vi "7118ValveCntrl.vi"() -> ()   [LabVIEW 2017]
doc: "Manually blink and LED attached to a digital output channel of a LINX device by clicking and LED control in LabVIEW."
uses:
  <vilib>/MakerHub/LINX/Public/Peripherals/Digital/Digital Write N Chans.vi
  <vilib>/MakerHub/LINX/Private/Local IO/LinxDigitalWrite.vi
  <vilib>/MakerHub/LINX/Public/Utilities/Check Channel.vi
  <vilib>/MakerHub/LINX/Public/Utilities/Open Serial.vi
  <vilib>/MakerHub/LINX/Private/Utilties/Generate Error.vi
  <vilib>/MakerHub/LINX/LMH-LINX.lvlib
panel:
  in  "Boolean":bool
  in  "device ID":u32 format="%.0x"
  in  "CHANNELS":u8[](array[numeric])
  out "Loop Rate (Hz)":u32
  in  "MANUAL CONTROLS":bool[](array[boolean])
  in  "Serial Port":refnum<visa-resource-name>
  in  "Stop Button":bool
  # "VALVE CONTROL\nVALVE CONTROl\nVALVE CONTROL\nVLV CNTRL"
  # "MCU Control"
  # "OPERATOR INSTRUCTIONS - MCU \n\n1. LOAD FIRMWARE ONTO MCU\n2. SELECT COM PORT\n3. SELECT ALL CHANNELS/CORRESPONDING TO MCU PIN NUMBERS\n4. RUN THE SCRIPT - WAIT 10-15 SECOND TO INITIALIZE  \n5. IF INITILIAZATION ERROR RECEIVED - RUN THE SCRIPT AGAIN\n6. CONTROLS ARE READY WHEN THE HZ RATE SETTLES"
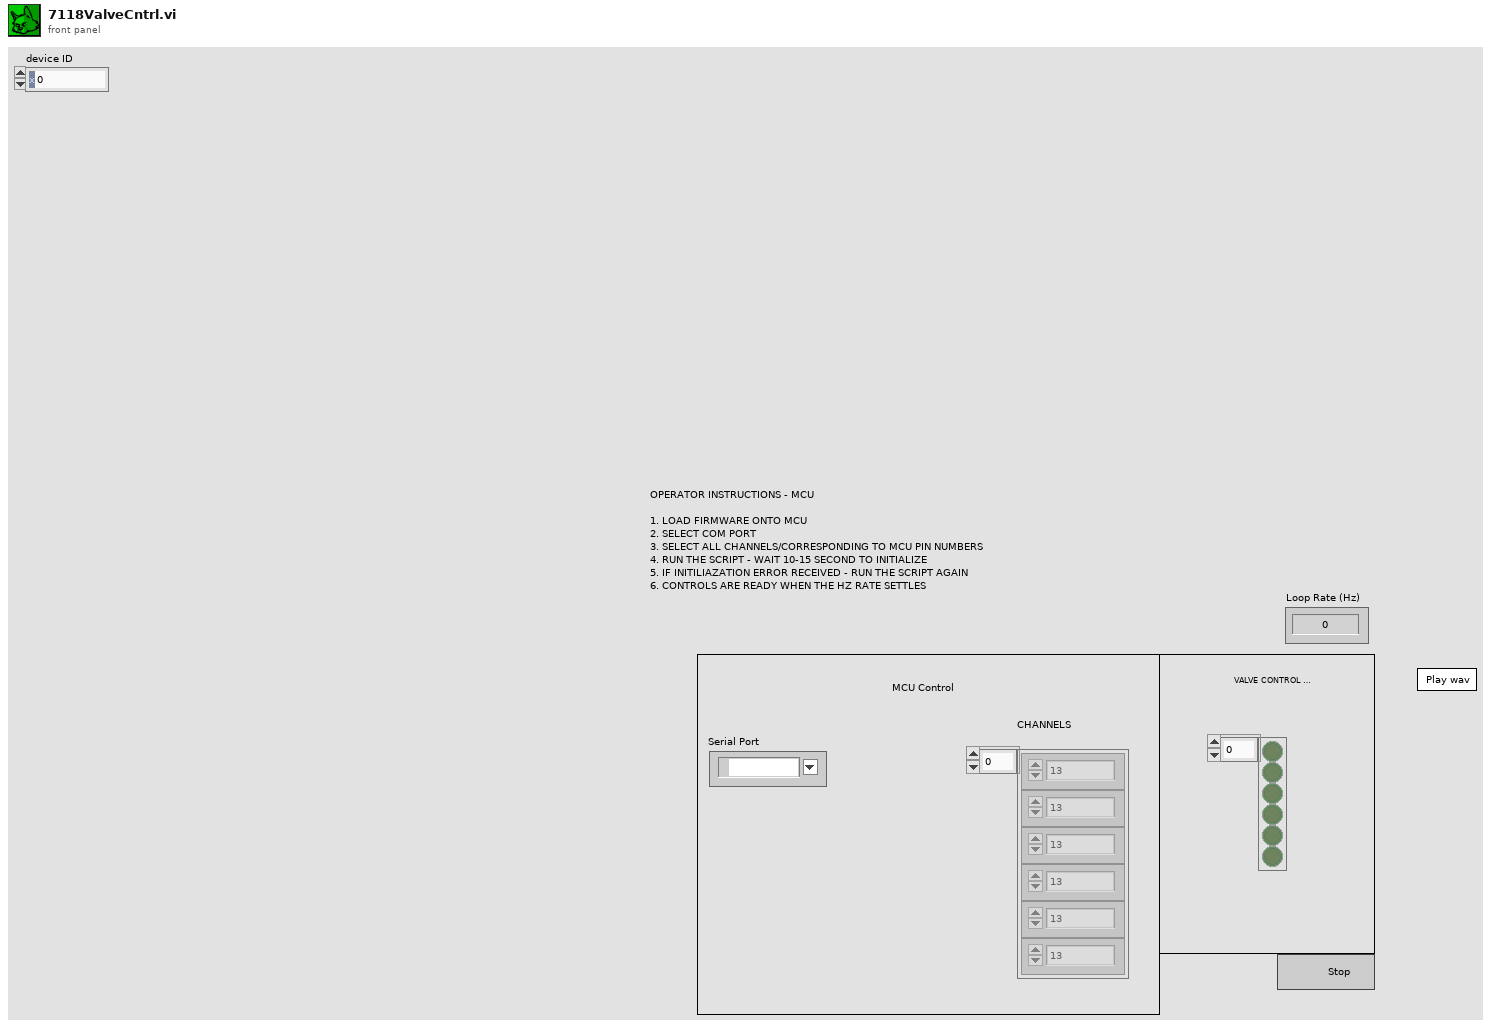
[diagram p1: front panel]
types:
  T1 = typedef "LMH-LINX.lvlib/LINX Ref.ctl" = cluster{"IO":T2, "Interface":T3, "LINX Device Config":T4}
  T2 = typedef "LMH-LINX.lvlib/Platform.ctl" = enum16{"Remote", "Local"}
  T3 = typedef "LMH-LINX.lvlib/Interface.ctl" = enum16{"Serial", "TCP"}
  T4 = typedef "LMH-LINX.lvlib/Device.lvlib/LINX Device Config.ctl" = cluster{"Interface":T3, "COM Port":refnum<visa-resource-name>, "TCP Configuration":T5, "Device Family":u8, "Device ID":u8, "Device Name":string, "TCP Ref":refnum<k5>, "Channels":T6}
  T5 = typedef "LMH-LINX.lvlib/Device.lvlib/TCP Config.ctl" = cluster{"IP Address":string, "Port":u16}
  T6 = typedef "LMH-LINX.lvlib/Channels.ctl" = cluster{"DI":u8[], "DO":u8[], "AI":u8[], "AO":u8[], "PWM":u8[], "QE":u8[], "UART":u8[], "I2C 2":u8[], "SPI":u8[], "CAN":u8[], "Servo":u8[], "AI Ref (V)":dbl, "AI Resolution (Bits)":u8, "AO Ref (V)":dbl, "AO Resolution (Bits)":u8}
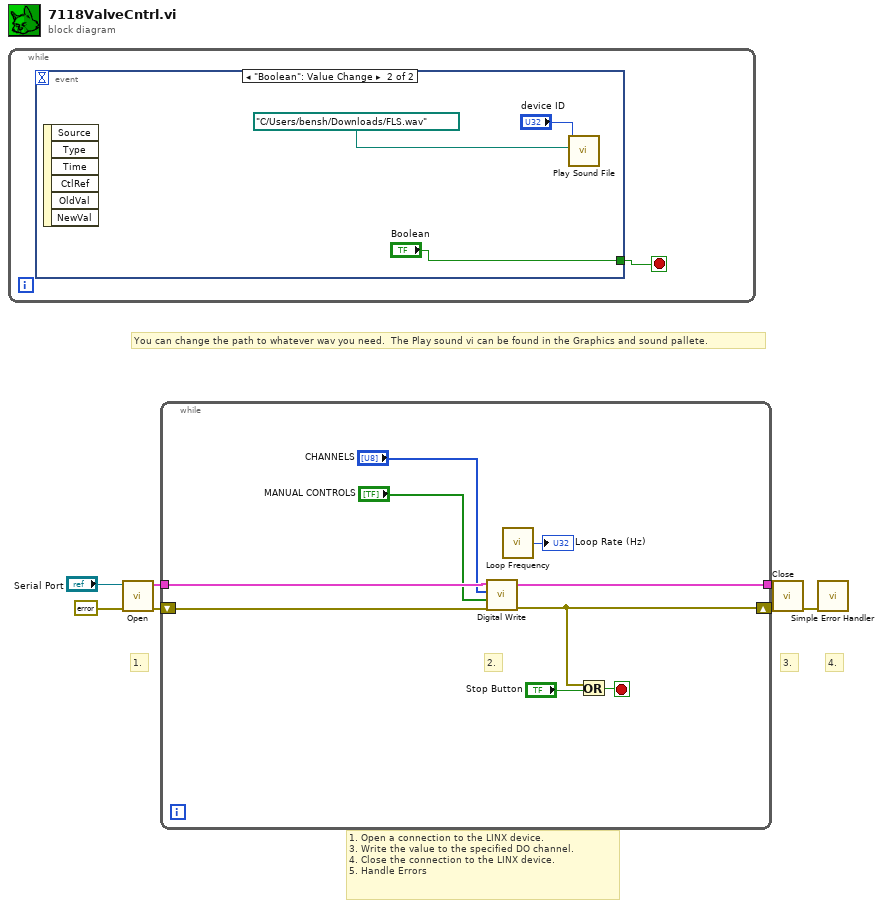
[diagram p0: block diagram]
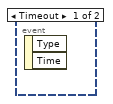
[diagram p2: hidden frame]
diagram:
  # "You can change the path to whatever wav you need.  The Play sound vi can be found in the Graphics and sound pallete."
  # "1. Open a connection to the LINX device.\n3. Write the value to the specified DO channel.\n4. Close the connection to the LINX device.\n5. Handle Errors"
  # "4."
  # "3."
  # "1."
  n1 = while {
    stop <- w8 stop-if-true
    n2 = event shown="[1] \"Boolean\": Value Change" {
      selector: _ -> [_ _]
      dyn-events: _ -> [_ _]
      timeout: _ -> [_ _]
      tunnel: [_ "Boolean"] -> w8
      event Timeout {
        n3 = event-data() -> ()  [unwired: 1 in, 2 out]
      }
      event "Boolean": Value Change {
        n4 = event-data() -> ()  [unwired: 1 in, 6 out]
        n5 = call <vilib>:"Play Sound File.vi"("path"=path "C:/Users/bensh/Downloads/FLS.wav", "device ID"="device ID") -> ()  [unwired: 8 in, 2 out]
      }
    }
  }
  n6 = call-poly <vilib>:"Open.vi"("Error In"=errorcluster {"status"=FALSE, "code"=0, "source"=""}, "Serial Port"="Serial Port") -> ("Error Out"=w6:errorcluster, "LINX Resource"=w7:T1)  [unwired: 7 in, 1 out]
  n7 = while {
    tunnel: w7 -> [w18]
    tunnel: [w17] -> w5
    shift-right: [w15] -> w4
    shift-left: w6 -> [w16]
    stop <- w20 stop-if-true
    # "2."
    n8 = call-poly <vilib>:"Digital Write.vi"("Error In"=w16, "Values"="MANUAL CONTROLS", "DO Channels"="CHANNELS", "LINX Resource"=w18) -> ("Error Out"=w15:errorcluster, "LINX Resource"=w17:T1)  [unwired: 6 in]
    n9 = call <vilib>:"Loop Frequency.vi"() -> ("Loop Rate (Hz)"=→"Loop Rate (Hz)":u32)
    n10 = Or(x=w15, y="Stop Button") -> (x .or. y?=w20:bool)
  }
  n11 = call <vilib>:"Close.vi"("Error In"=w4, "LINX Resource"=w5) -> ("Error Out"=w2:errorcluster)  [unwired: 9 in]
  n12 = call <vilib>:"Simple Error Handler.vi"("error in (no error)"=w2) -> ()  [unwired: 4 in, 5 out]
